vi "Read Variable Value.vi"(8 "error in (no error)":errorcluster, 9 "Default Value":string, 10 "String":string, 11 "Variant in":variant) -> (0 "error out":errorcluster, 1 "Value":string, 2 "Found":bool, 3 "Variant out":variant)   [LabVIEW 2020, in "CSMStand(Lite).lvlib"]
uses:
  CSMStand(Lite).lvlib
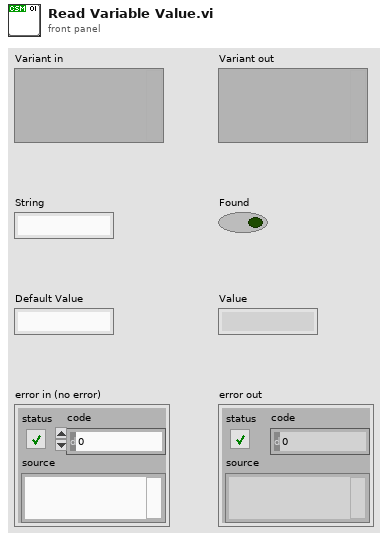
[diagram p1: front panel]
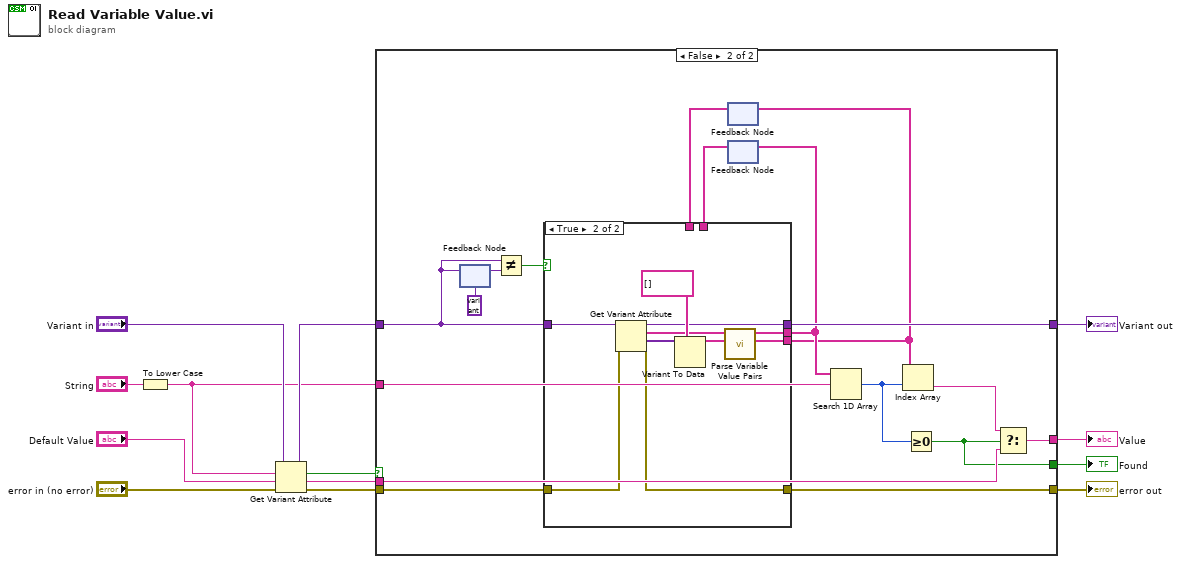
[diagram p0: block diagram]
diagram:
  n1 = To Lower Case(string="String") -> (all lower case string=w1:string)
  n2 = Get Variant Attribute(Variant="Variant in", name=w1, default value (empty Variant)="Default Value") -> (duplicate Variant=w5:variant, found=w2:bool, value=w3:string)  [unwired: 1 in, 1 out]
  n3 = case shown="False" w2 {
    selector: w2 -> [w14 _]
    tunnel: [w16 w30] -> w12
    tunnel: [w13 w24] -> w11
    tunnel: [w14 w23] -> w10
    tunnel: [w15 w32] -> w9
    tunnel: "error in (no error)" -> [w16 w33]
    tunnel: w5 -> [w15 w29]
    tunnel: w3 -> [w13 w25]
    tunnel: w1 -> [_ w31]
    frame True {
    }
    frame False {
      n4 = feedback-in #1(w29) -> ()
      n5 = feedback #1(variant) -> (w28:variant)
      n6 = Not Equal?(x=w29, y=w28) -> (x != y?=w22:bool)
      n7 = feedback #2() -> (w17:string[])  [unwired: 1 in]
      n8 = feedback #3() -> (w19:string[])  [unwired: 1 in]
      n9 = case shown="True" w22 {
        tunnel: w33 -> [w37 w47]
        tunnel: [w36 w42] -> w32
        tunnel: [w35 w41] -> w20
        tunnel: [w34 w40] -> w18
        tunnel: [w37 w39] -> w30
        tunnel: w29 -> [w36 w38]
        tunnel: w19 -> [w35 _]
        tunnel: w17 -> [w34 _]
        frame False {
        }
        frame True {
          n10 = Get Variant Attribute(Variant=w38, error in=w47) -> (duplicate Variant=w42:variant, names=w44:string[], values=w46:variant[], error out=w39:errorcluster)  [unwired: 2 in]
          n11 = Variant To Data(type=string[] [] ("String 2"), Variant=w46) -> (data=w43:string[])  [unwired: 1 in, 1 out]
          n12 = call "Parse Variable Value Pairs.vi"("Value"=w43, "Name"=w44) -> ("Value"=w40:string[], "Name2"=w41:string[])  [unwired: 8 in]
        }
      }
      n13 = feedback-in #2(w18) -> ()
      n14 = feedback-in #3(w20) -> ()
      n15 = Search 1D Array(1D array=w20, element=w31) -> (index of element=w27:i32)  [unwired: 1 in]
      n16 = Index Array(array=w18, index=w27) -> (element=w26:string)
      n17 = Greater Or Equal To 0?(x=w27) -> (x >= 0?=w23:bool)
      n18 = Select(t=w26, s=w23, f=w25) -> (s? t:f=w24:string)
    }
  }
  "error out" <- w12
  "Value" <- w11
  "Found" <- w10
  "Variant out" <- w9
